vi "S3-SenseBall.vi"(5 "Harvester Speed":dbl, 7 "Conveyor Speed":dbl, 8 "Shoot":bool, 9 "Sense Ball":bool, 11 "Ball S3 Process":bool) -> (0 "Conveyer Output":dbl, 1 "Ball S3 Process Output":bool, 2 "Shoot Output":bool, 3 "Ball Counter":dbl)   [LabVIEW 2011]
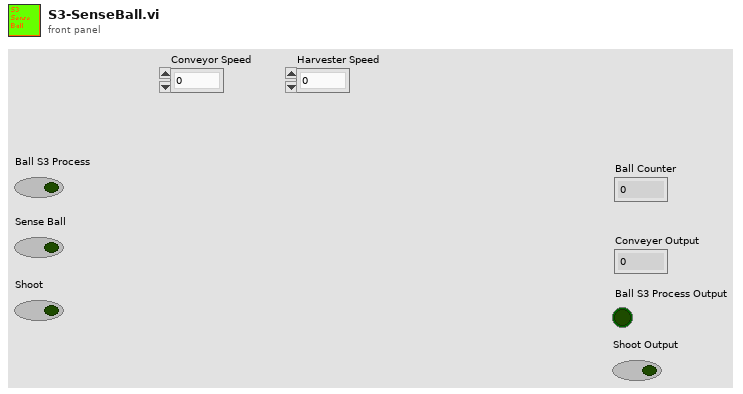
[diagram p1: front panel]
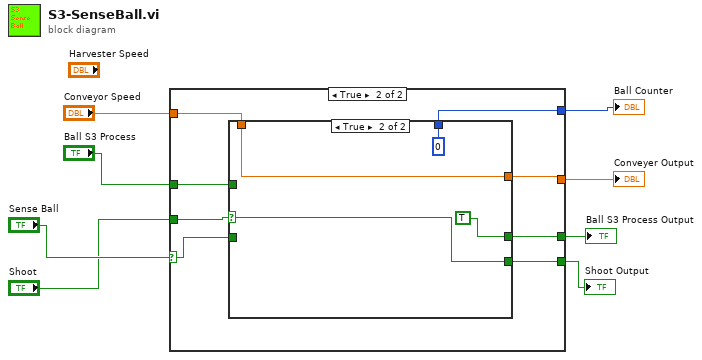
[diagram p0: block diagram]
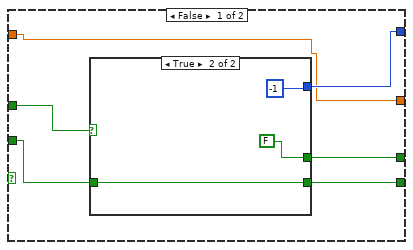
[diagram p2: hidden frame]
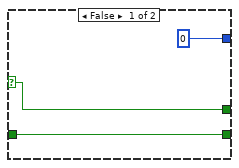
[diagram p3: hidden frame]
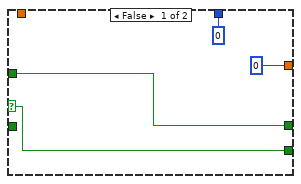
[diagram p4: hidden frame]
diagram:
  n1 = case shown="True" "Sense Ball" {
    selector: "Sense Ball" -> [_ w26]
    tunnel: [w9 w27] -> w7
    tunnel: "Shoot" -> [w11 w28]
    tunnel: [w12 w25] -> w5
    tunnel: "Ball S3 Process" -> [w14 w22]
    tunnel: [w13 w24] -> w3
    tunnel: [w10 w23] -> w2
    tunnel: "Conveyor Speed" -> [w9 w21]
    frame False {
      n2 = case shown="True" w14 {
        selector: w14 -> [w16 _]
        tunnel: [w15 w18] -> w13
        tunnel: [0 -1] -> w12
        tunnel: w11 -> [w15 w18]
        tunnel: [w16 FALSE] -> w10
        frame False {
        }
        frame True {
        }
      }
    }
    frame True {
      n3 = case shown="True" w28 {
        selector: w28 -> [w30 w33]
        tunnel: [0 w35] -> w27
        tunnel: w26 -> [_ _]
        tunnel: [0 0] -> w25
        tunnel: [w30 w33] -> w24
        tunnel: [w29 TRUE] -> w23
        tunnel: w22 -> [w29 _]
        tunnel: w21 -> [_ w35]
        frame False {
        }
        frame True {
        }
      }
    }
  }
  "Conveyer Output" <- w7
  "Ball Counter" <- w5
  "Ball S3 Process Output" <- w2
  "Shoot Output" <- w3
